vi "Read Example With Events (advanced).vi"(11 "Error In":errorcluster) -> (15 "Error Out":errorcluster)   [LabVIEW 2016]
uses:
  LabVIEW_GEA2_Toolkit.lvlibp/type defs/Data In.ctl
  LabVIEW_GEA2_Toolkit.lvlibp
panel:
  out "Log":string
  in  "Input Data":T1={"Source"=228, "Destination"=0, "Command"=0, "Message"=""} {"Command" format="%02x"; "Destination" format="%02x"; "Source" format="%02x"}
  in  "Stop":bool
  in  "Send":bool
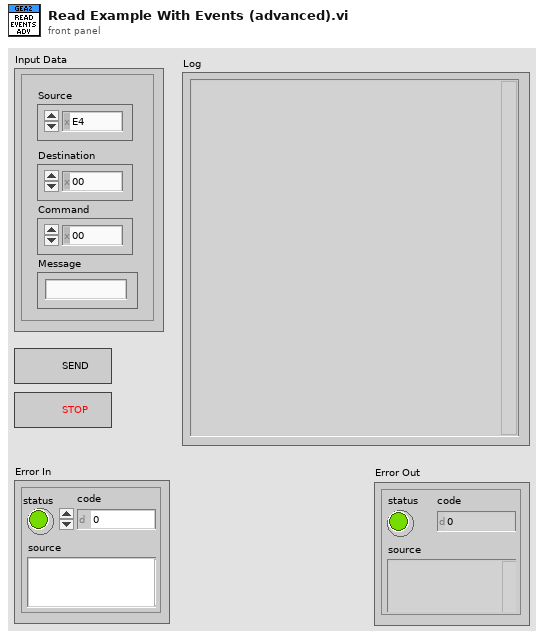
[diagram p1: front panel]
types:
  T1 = typedef "LabVIEW_GEA2_Toolkit.lvlibp/Data In.ctl" = cluster{"Source":u8, "Destination":u8, "Command":u8, "Message":string}
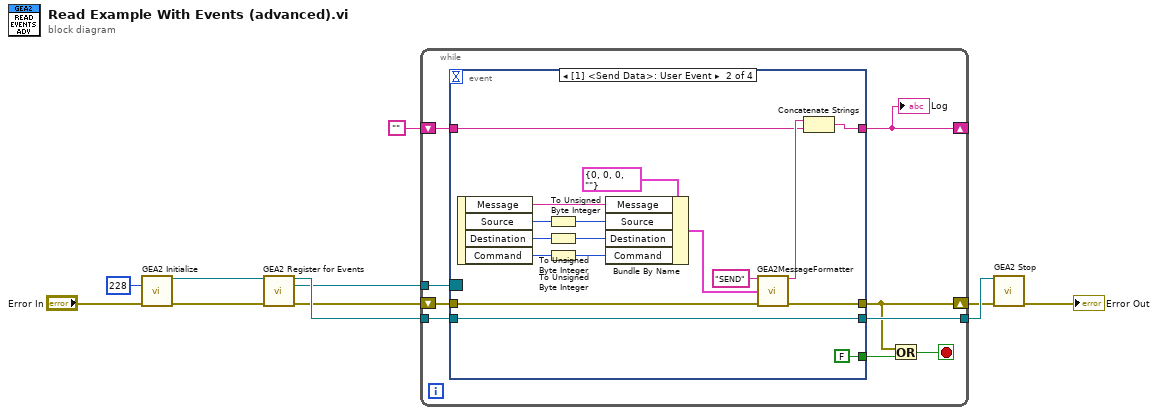
[diagram p0: block diagram]
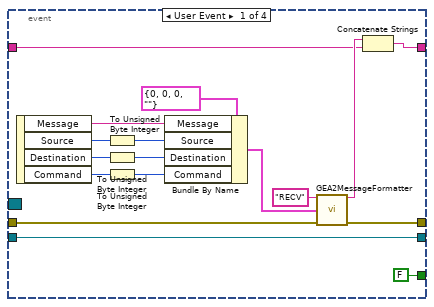
[diagram p2: hidden frame]
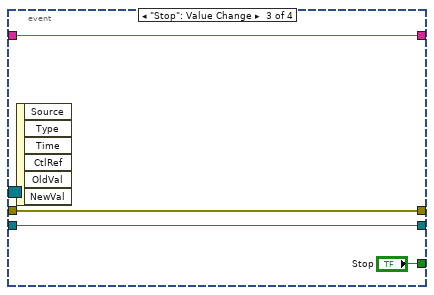
[diagram p3: hidden frame]
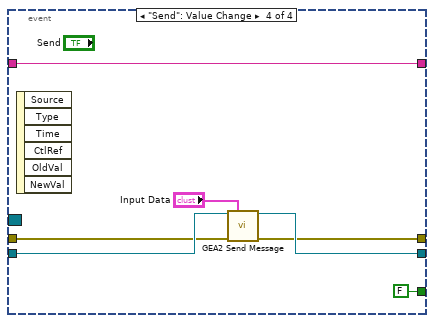
[diagram p4: hidden frame]
diagram:
  n1 = call "GEA2 Initialize.vi"("Source Address"=u8 228, "error in"="Error In") -> ("GEA2 Reference Out"=w9:refnum<k24>, "error out"=w10:errorcluster)  [unwired: 11 in, 1 out]
  n2 = call "GEA2 Register for Events.vi"("GEA2 Reference In"=w9, "Error In"=w10) -> ("GEA2 Reference Out"=w5:refnum<k24>, "Event Registration Refnum"=w3:refnum<event-registration>, "Error Out"=w4:errorcluster)  [unwired: 11 in]
  n3 = while {
    tunnel: w3 -> [w19]
    tunnel: [w16] -> w8
    tunnel: w5 -> [w17]
    shift-right: [w15] -> w7
    shift-left: w4 -> [w18]
    shift-right: [w13] -> _
    shift-left: "" -> [w14]
    stop <- w20 stop-if-true
    n4 = event shown="[1] <Send Data>: User Event" {
      selector: w19 -> [_ _ _ _]
      dyn-events: _ -> [_ _ _ _]
      timeout: _ -> [_ _ _ _]
      tunnel: w18 -> [w27 w44 w56 w63]
      tunnel: [w26 w43 w56 w62] -> w15
      tunnel: w17 -> [w25 w42 w57 w65]
      tunnel: [w25 w42 w57 w64] -> w16
      tunnel: w14 -> [w21 w38 w55 w60]
      tunnel: [w24 w41 w55 w60] -> w13
      tunnel: [FALSE ("Stop") FALSE ("Stop") "Stop" FALSE ("Stop")] -> w12
      event User Event {
        n5 = event-data() -> ("Message"=w31:string, "Source"=w32:u8, "Destination"=w33:u8, "Command"=w34:u8)  [unwired: 1 in]
        n6 = To Unsigned Byte Integer(number=w32) -> (unsigned 8bit integer=w36:u8)
        n7 = To Unsigned Byte Integer(number=w33) -> (unsigned 8bit integer=w37:u8)
        n8 = To Unsigned Byte Integer(number=w34) -> (unsigned 8bit integer=w35:u8)
        n9 = Bundle By Name(cluster=T1 {"Source"=0, "Destination"=0, "Command"=0, "Message"=""} ("GEA2 Data In"), "Message"=w31, "Source"=w36, "Destination"=w37, "Command"=w35) -> (w29:T1)
        n10 = call "GEA2MessageFormatter.vi"("Prefix(Send/Recv)"="RECV", "GEA2 Data In"=w29, "Error In"=w27) -> ("Output String"=w22:string, "Error Out"=w26:errorcluster)  [unwired: 11 in]
        n11 = Concatenate Strings(w22, w21) -> (w24:string)
      }
      event User Event {
        n12 = event-data() -> ("Message"=w48:string, "Source"=w49:u8, "Destination"=w50:u8, "Command"=w51:u8)  [unwired: 1 in]
        n13 = To Unsigned Byte Integer(number=w49) -> (unsigned 8bit integer=w53:u8)
        n14 = To Unsigned Byte Integer(number=w50) -> (unsigned 8bit integer=w54:u8)
        n15 = To Unsigned Byte Integer(number=w51) -> (unsigned 8bit integer=w52:u8)
        n16 = Bundle By Name(cluster=T1 {"Source"=0, "Destination"=0, "Command"=0, "Message"=""} ("GEA2 Data In"), "Message"=w48, "Source"=w53, "Destination"=w54, "Command"=w52) -> (w46:T1)
        n17 = call "GEA2MessageFormatter.vi"("Prefix(Send/Recv)"="SEND", "GEA2 Data In"=w46, "Error In"=w44) -> ("Output String"=w39:string, "Error Out"=w43:errorcluster)  [unwired: 11 in]
        n18 = Concatenate Strings(w39, w38) -> (w41:string)
      }
      event "Stop": Value Change {
        n19 = event-data() -> ()  [unwired: 1 in, 6 out]
      }
      event "Send": Value Change {
        n20 = event-data() -> ()  [unwired: 1 in, 6 out]
        n21 = call "GEA2 Send Message.vi"("GEA2 Reference In"=w65, "Input Data"="Input Data", "Error In"=w63) -> ("GEA2 Reference Out"=w64:refnum<k24>, "Error Out"=w62:errorcluster)  [unwired: 11 in]
      }
    }
    "Log" <- w13
    n22 = Or(x=w15, y=w12) -> (x .or. y?=w20:bool)
  }
  n23 = call "GEA2 Stop.vi"("GEA2 Reference In"=w8, "Error In"=w7) -> ("Error Out"=→"Error Out":errorcluster)  [unwired: 13 in]
